vi "Update.vi"(8 "error in (no error)":errorcluster, 11 "GameObject in":refnum<class "GameObject.lvclass">) -> (0 "error out":errorcluster, 3 "GameObject out":refnum<class "GameObject.lvclass">)   [LabVIEW 2019, in "RT_Game.lvlib" / "GameObject.lvclass"]
uses:
  GameObject.lvclass
  GameObject.lvclass/GameObject.ctl
  Globals.vi
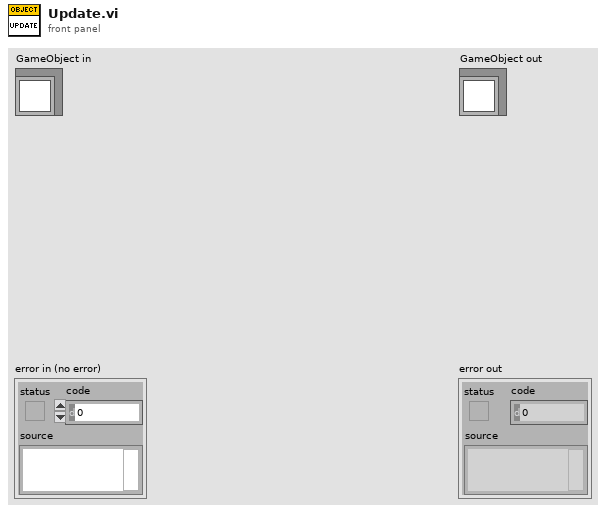
[diagram p1: front panel]
types:
  T1 = typedef "Velocity.ctl" = cluster{"x":dbl, "y":dbl}
  T2 = typedef "RT_Game.lvlib/Game.lvclass/Coordinate.ctl" = cluster{"x":dbl, "y":dbl}
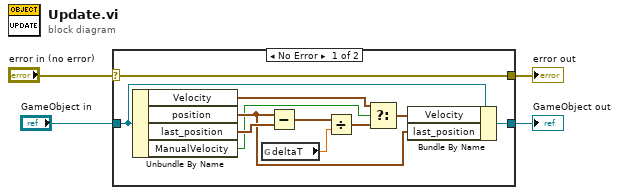
[diagram p0: block diagram]
diagram:
  n1 = case shown="No Error" "error in (no error)" {
    selector: "error in (no error)" -> [w15 w17]
    tunnel: [w15 w17] -> w3
    tunnel: [w14 w16] -> w1
    tunnel: "GameObject in" -> [w13 w16]
    frame No Error {
      n2 = Unbundle By Name(w13) -> ("Velocity"=w6:T1, "position"=w11:T2, "last_position"=w12:T2, "ManualVelocity"=w5:bool)
      n3 = global read "Globals.vi" "deltaT"() -> (w9:dbl)
      n4 = Subtract(x=w11, y=w12) -> (x-y=w10:T2)
      n5 = Divide(x=w10, y=w9) -> (x/y=w7:T2)
      n6 = Select(t=w6, s=w5, f=w7) -> (s? t:f=w8:T2)
      n7 = Bundle By Name(cluster=w13, "Velocity"=w8, "last_position"=w11) -> (w14:refnum<class "GameObject.lvclass">)
    }
    frame Error {
    }
  }
  "error out" <- w3
  "GameObject out" <- w1
